vi "sint64 decode.vi"(11 "zigzag64":u64) -> (3 "sint64":i64)   [LabVIEW 2013, in "protocol buffers encoder.lvlib"]
uses:
  protocol buffers encoder.lvlib
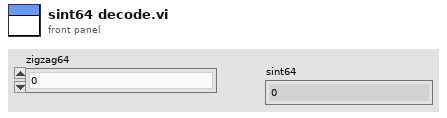
[diagram p1: front panel]
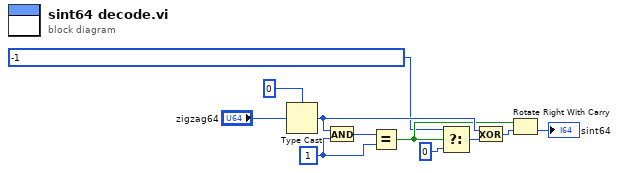
[diagram p0: block diagram]
diagram:
  w10 = i64 1 ("y")
  n1 = Type Cast(type=i64 0 ("y"), x="zigzag64") -> (*(type *) &x=w8:i64)
  n2 = And(x=w8, y=w10) -> (x .and. y?=w11:i64)
  n3 = Equal?(x=w11, y=w10) -> (x = y?=w5:bool)
  n4 = Select(t=i64 -1 ("y"), s=w5, f=i64 0 ("t")) -> (s? t:f=w9:i64)
  n5 = Exclusive Or(1:w9, 2:w8) -> (0:w6:i64)
  n6 = Rotate Right With Carry(2:w6, 3:w5) -> (0:→"sint64":i64)  [unwired: 1 out]
